vi "Main -- separate writes.vi"() -> ()   [LabVIEW 2013]
uses:
  <vilib>/myRIO/Instrument Drivers/Onboard IO/I2C/typedefs/I2C User Configuration.ctl
  <vilib>/myRIO/Instrument Drivers/Onboard IO/I2C/typedefs/I2C Transfer Rate.ctl
  <vilib>/myRIO/Common/Instrument Driver Framework/myRIO v1.0/I2C/vis/myRIO v1.1 Open I2C.vi
  <vilib>/myRIO/Common/Instrument Driver Framework/myRIO v1.0/UART/vis/myRIO v1.0 Close UART.vi
  <vilib>/myRIO/Common/Instrument Driver Framework/Utilities/vis/Validate Channels.vi
  <vilib>/myRIO/Common/Instrument Driver Framework/myRIO v1.0/I2C/vis/myRIO v1.0 Reserve I2C.vi
  <vilib>/myRIO/Common/Instrument Driver Framework/myRIO v1.0/I2C/vis/myRIO v1.0 Build MUX Configuration I2C.vi
  <vilib>/myRIO/Common/Instrument Driver Framework/myRIO v1.0/Resource Manager/vis/myRIO v1.0 Reserve Channel List.vi
  <vilib>/myRIO/Common/Instrument Driver Framework/myRIO v1.0/Resource Manager/vis/myRIO v1.0 Create Configuration List.vi
  <vilib>/myRIO/Common/Instrument Driver Framework/myRIO v1.0/Resource Manager/vis/myRIO v1.0 Reserve Channel.vi
  <vilib>/myRIO/Common/Instrument Driver Framework/myRIO v1.0/Resource Manager/vis/myRIO v1.0 Unreserve Channel.vi
  <vilib>/myRIO/Common/Instrument Driver Framework/myRIO v1.0/Resource Manager/vis/myRIO v1.0 Build Mutex Name.vi
  <vilib>/myRIO/Common/Instrument Driver Framework/myRIO v1.0/myRIO v1.1 Open.vi
  <vilib>/Utility/VariantDataType/GetNumericInfo.vi
  <vilib>/Utility/error.llb/Error Cluster From Error Code.vi
  <vilib>/myRIO/Common/Instrument Driver Framework/Utilities/vis/IO Manager.vi
  <vilib>/myRIO/Common/Instrument Driver Framework/Utilities/vis/Configuration Manager.vi
  <vilib>/myRIO/Common/Instrument Driver Framework/myRIO v1.0/Resource Manager/vis/myRIO v1.0 Configure IO.vi
  <vilib>/myRIO/Common/Instrument Driver Framework/myRIO v1.0/myRIO v1.0 Close.vi
  <vilib>/myRIO/Common/Instrument Driver Framework/myRIO v1.0/I2C/vis/myRIO v1.0 Configure I2C.vi
  <vilib>/myRIO/Common/Instrument Driver Framework/myRIO v1.0/I2C/vis/myRIO v1.0 Write I2C.vi
  <vilib>/myRIO/Common/Instrument Driver Framework/myRIO v1.0/I2C/vis/myRIO v1.0 Read I2C.vi
  <vilib>/myRIO/Common/Instrument Driver Framework/Utilities/vis/FPGA Ref Manager.vi
  <vilib>/myRIO/Common/Instrument Driver Framework/myRIO v1.0/myRIO v1.0 Reset FPGA.vi
  <vilib>/myRIO/Instrument Drivers/Utilities/Utilities.lvlib
  <vilib>/myRIO/Instrument Drivers/Onboard IO/I2C/I2C.lvlib
panel:
  out "INT_SOURCE register":bool[](array[boolean])
  out "Waveform Chart":cluster{i16, i16, i16}(graph)
  out "Bytes":u8[](array[numeric]) format="%x"
  out "Z":i16
  out "Y":i16
  out "X":i16
  in  "[ESC]":bool
  # "Accelerometer demo"
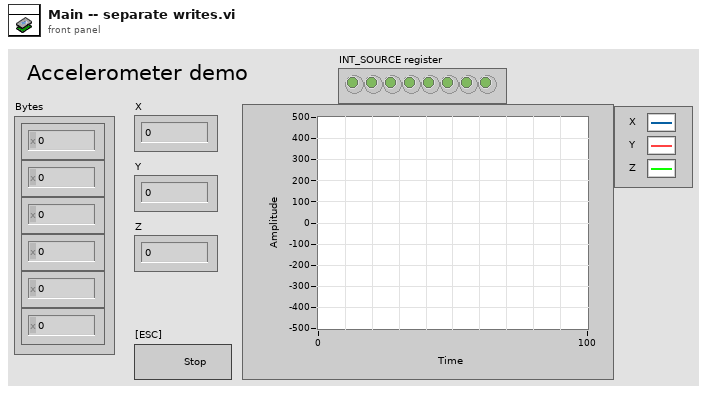
[diagram p1: front panel]
types:
  T1 = typedef "I2C.lvlib/I2C User Configuration.ctl" = cluster{"I2C Transfer Rate":T2}
  T2 = typedef "I2C.lvlib/I2C Transfer Rate.ctl" = enum16{"Standard Mode (100 kbps)", "Fast Mode (400 kbps)"}
  T3 = typedef "I2C.lvlib/I2C Reference.ctl" = cluster{"myRIO Reference":T4, "I2C Channels Enum":T8, "I2C Configuration":T9}
  T4 = typedef "myRIO Generic Hardware Reference.ctl" = cluster{"myRIO Model":T5, "myRIO Hardware Reference":T6}
  T5 = typedef "Hardware Version Enum.ctl" = enum16{"Unknown", "myRIO-1900", "myRIO-1950"}
  T6 = typedef "myRIO v1.0 Reference.ctl" = cluster{"Generic FPGA Reference":T7, "Allow multiple opens":bool}
  T7 = typedef "Generic FPGA Reference.ctl" = refnum<k20>
  T8 = typedef "I2C Channels Enum.ctl" = enum16{"Not Connected", "A/I2C", "B/I2C"}
  T9 = typedef "I2C.lvlib/I2C Configuration.ctl" = cluster{"I2C Transfer Rate":T2}
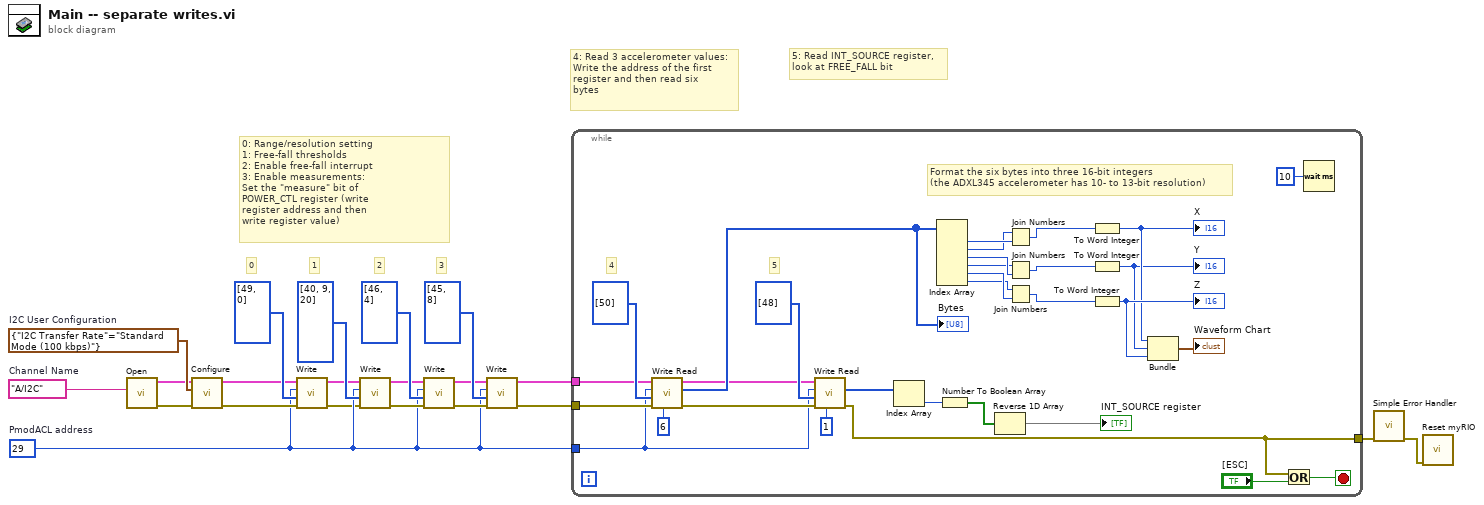
[diagram p0: block diagram]
diagram:
  w18 = T1 {"I2C Transfer Rate"=enum."Standard Mode (100 kbps)"}  # I2C User Configuration
  w19 = tag "A/I2C"  # Channel Name
  w3 = u8 29  # PmodACL address
  # "0"
  # "5: Read INT_SOURCE register,\nlook at FREE_FALL bit"
  # "4: Read 3 accelerometer values:\nWrite the address of the first\nregister and then read six\nbytes"
  # "3"
  # "2"
  # "1"
  # "0: Range/resolution setting\n1: Free-fall thresholds\n2: Enable free-fall interrupt\n3: Enable measurements:\nSet the \"measure\" bit of\nPOWER_CTL register (write\nregister address and then\nwrite register value)"
  n1 = call <vilib>:"Open.vi"("Channel Name"=w19) -> ("error out"=w16:errorcluster, "I2C Ref Out"=w17:T3)  [unwired: 9 in]
  n2 = call <vilib>:"Configure.vi"("error in (no error)"=w16, "I2C User Configuration"=w18, "I2C Ref In"=w17) -> ("error out"=w4:errorcluster, "I2C Ref Out"=w5:T3)  [unwired: 7 in]
  n3 = call <vilib>:"Write.vi"("error in (no error)"=w4, "Bytes to Write"=u8[] [49, 0], "Slave Address (7-bit)"=w3, "I2C Ref In"=w5) -> ("error out"=w1:errorcluster, "I2C Ref Out"=w2:T3)  [unwired: 6 in]
  n4 = call <vilib>:"Write.vi"("error in (no error)"=w1, "Bytes to Write"=u8[] [40, 9, 20], "Slave Address (7-bit)"=w3, "I2C Ref In"=w2) -> ("error out"=w9:errorcluster, "I2C Ref Out"=w10:T3)  [unwired: 6 in]
  n5 = call <vilib>:"Write.vi"("error in (no error)"=w9, "Bytes to Write"=u8[] [46, 4], "Slave Address (7-bit)"=w3, "I2C Ref In"=w10) -> ("error out"=w7:errorcluster, "I2C Ref Out"=w8:T3)  [unwired: 6 in]
  n6 = call <vilib>:"Write.vi"("error in (no error)"=w7, "Bytes to Write"=u8[] [45, 8], "Slave Address (7-bit)"=w3, "I2C Ref In"=w8) -> ("error out"=w14:errorcluster, "I2C Ref Out"=w13:T3)  [unwired: 6 in]
  n7 = while {
    tunnel: [w28] -> w20
    tunnel: w3 -> [w26]
    tunnel: w14 -> [w40]
    tunnel: w13 -> [w39]
    stop <- w51 stop-if-true
    # "5"
    # "4"
    # "Format the six bytes into three 16-bit integers\n(the ADXL345 accelerometer has 10- to 13-bit resolution)"
    n8 = call <vilib>:"Write Read.vi"("Byte Count"=u32 6, "error in (no error)"=w40, "Bytes to Write"=u8[] [50], "Slave Address (7-bit)"=w26, "I2C Ref In"=w39) -> ("error out"=w27:errorcluster, "Bytes Read"=w32:u8[], "I2C Ref Out"=w29:T3)  [unwired: 3 in]
    "Bytes" <- w32
    n9 = call <vilib>:"Write Read.vi"("Byte Count"=u32 1, "error in (no error)"=w27, "Bytes to Write"=u8[] [48], "Slave Address (7-bit)"=w26, "I2C Ref In"=w29) -> ("error out"=w28:errorcluster, "Bytes Read"=w25:u8[])  [unwired: 3 in, 1 out]
    n10 = Index Array "Index Array"(array=w25) -> (element=w24:u8)  [unwired: 1 in]
    n11 = Index Array "Index Array"(array=w32) -> (element #1=w38:u8, element #2=w37:u8, element #3=w36:u8, element #4=w35:u8, element #5=w34:u8, element #6=w33:u8)  [unwired: 6 in]
    n12 = Number To Boolean Array(number=w24) -> (Boolean array=w23:bool[])
    n13 = Reverse 1D Array(array=w23) -> (reversed array=→"INT_SOURCE register":bool[])
    n14 = Join Numbers(hi=w37, lo=w38) -> ((hi.lo)=w49:u16)
    n15 = Join Numbers(hi=w35, lo=w36) -> ((hi.lo)=w48:u16)
    n16 = Join Numbers(hi=w33, lo=w34) -> ((hi.lo)=w47:u16)
    n17 = To Word Integer(number=w49) -> (16bit integer=w44:i16)
    "X" <- w44
    n18 = To Word Integer(number=w48) -> (16bit integer=w43:i16)
    "Y" <- w43
    n19 = To Word Integer(number=w47) -> (16bit integer=w46:i16)
    "Z" <- w46
    n20 = Bundle "Bundle"(w44, w43, w46) -> (→"Waveform Chart":cluster{i16, i16, i16})  [unwired: 1 in]
    n21 = Or(x=w28, y="[ESC]") -> (x .or. y?=w51:bool)
    n22 = Wait (ms)(milliseconds to wait=u32 10) -> ()  [unwired: 1 out]
  }
  n23 = call <vilib>:"Simple Error Handler.vi"("error in (no error)"=w20) -> ("error out"=w21:errorcluster)  [unwired: 4 in, 4 out]
  n24 = call <vilib>:"Reset myRIO.vi"("error in (no error)"=w21) -> ()  [unwired: 10 in, 1 out]
